vi "INTELLIFAUCET Need Adjustment PID.vi"(1 "GPM reading":dbl, 4 "GPM Target(3)":dbl, 5 "Error In":errorcluster, 10 "State":T1, 12 "TEMP,FLOW":T2=enum."FLOW") -> (13 "PI Output":dbl, 17 "Control Variable (Temp/GPM) Output":dbl, 18 "Micro Amp":i32, 19 "Error Out":errorcluster)   [LabVIEW 2023]
uses:
  Type Definitions/INTELLIFAUCT Temp Flow.ctl
  Type Definitions/HEWH Purge Draw.ctl
  <vilib>/addons/control/pid/NI_PID_autopid.lvlib
panel:
  in  "MV1:":dbl(slide)=15.081495361740814 scale=-100.0..100.0
  # "1.019811"
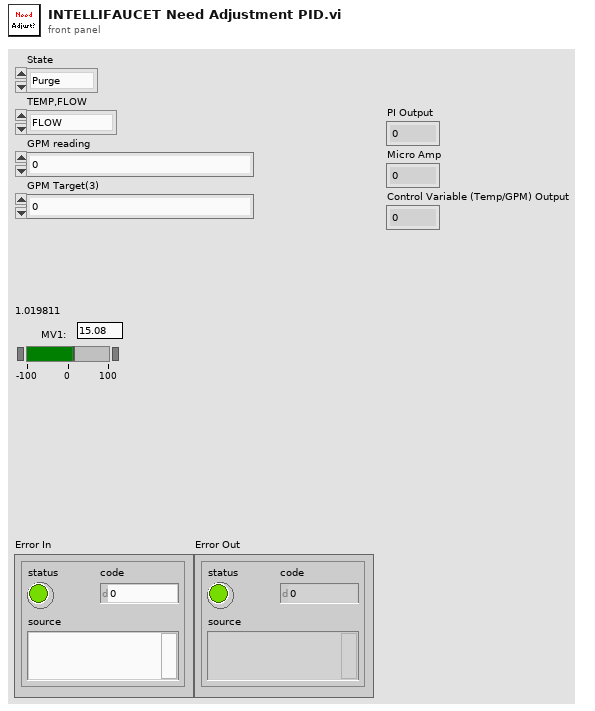
[diagram p1: front panel]
types:
  T1 = typedef "HEWH Purge Draw.ctl" = enum16{"Purge", "Draw"}
  T2 = typedef "INTELLIFAUCT Temp Flow.ctl" = enum8{"TEMP", "FLOW", "Prop Valve"}
  T3 = cluster{"process gain":dbl, "time constant (s)":dbl, "delay time (s)":dbl}
  T4 = cluster{"type of controller":u16, "time constant factor":dbl, "step amplitude":dbl}
  T5 = cluster{"proportional gain (Kc)":dbl, "integral time (Ti, min)":dbl, "derivative time (Td, min)":dbl}
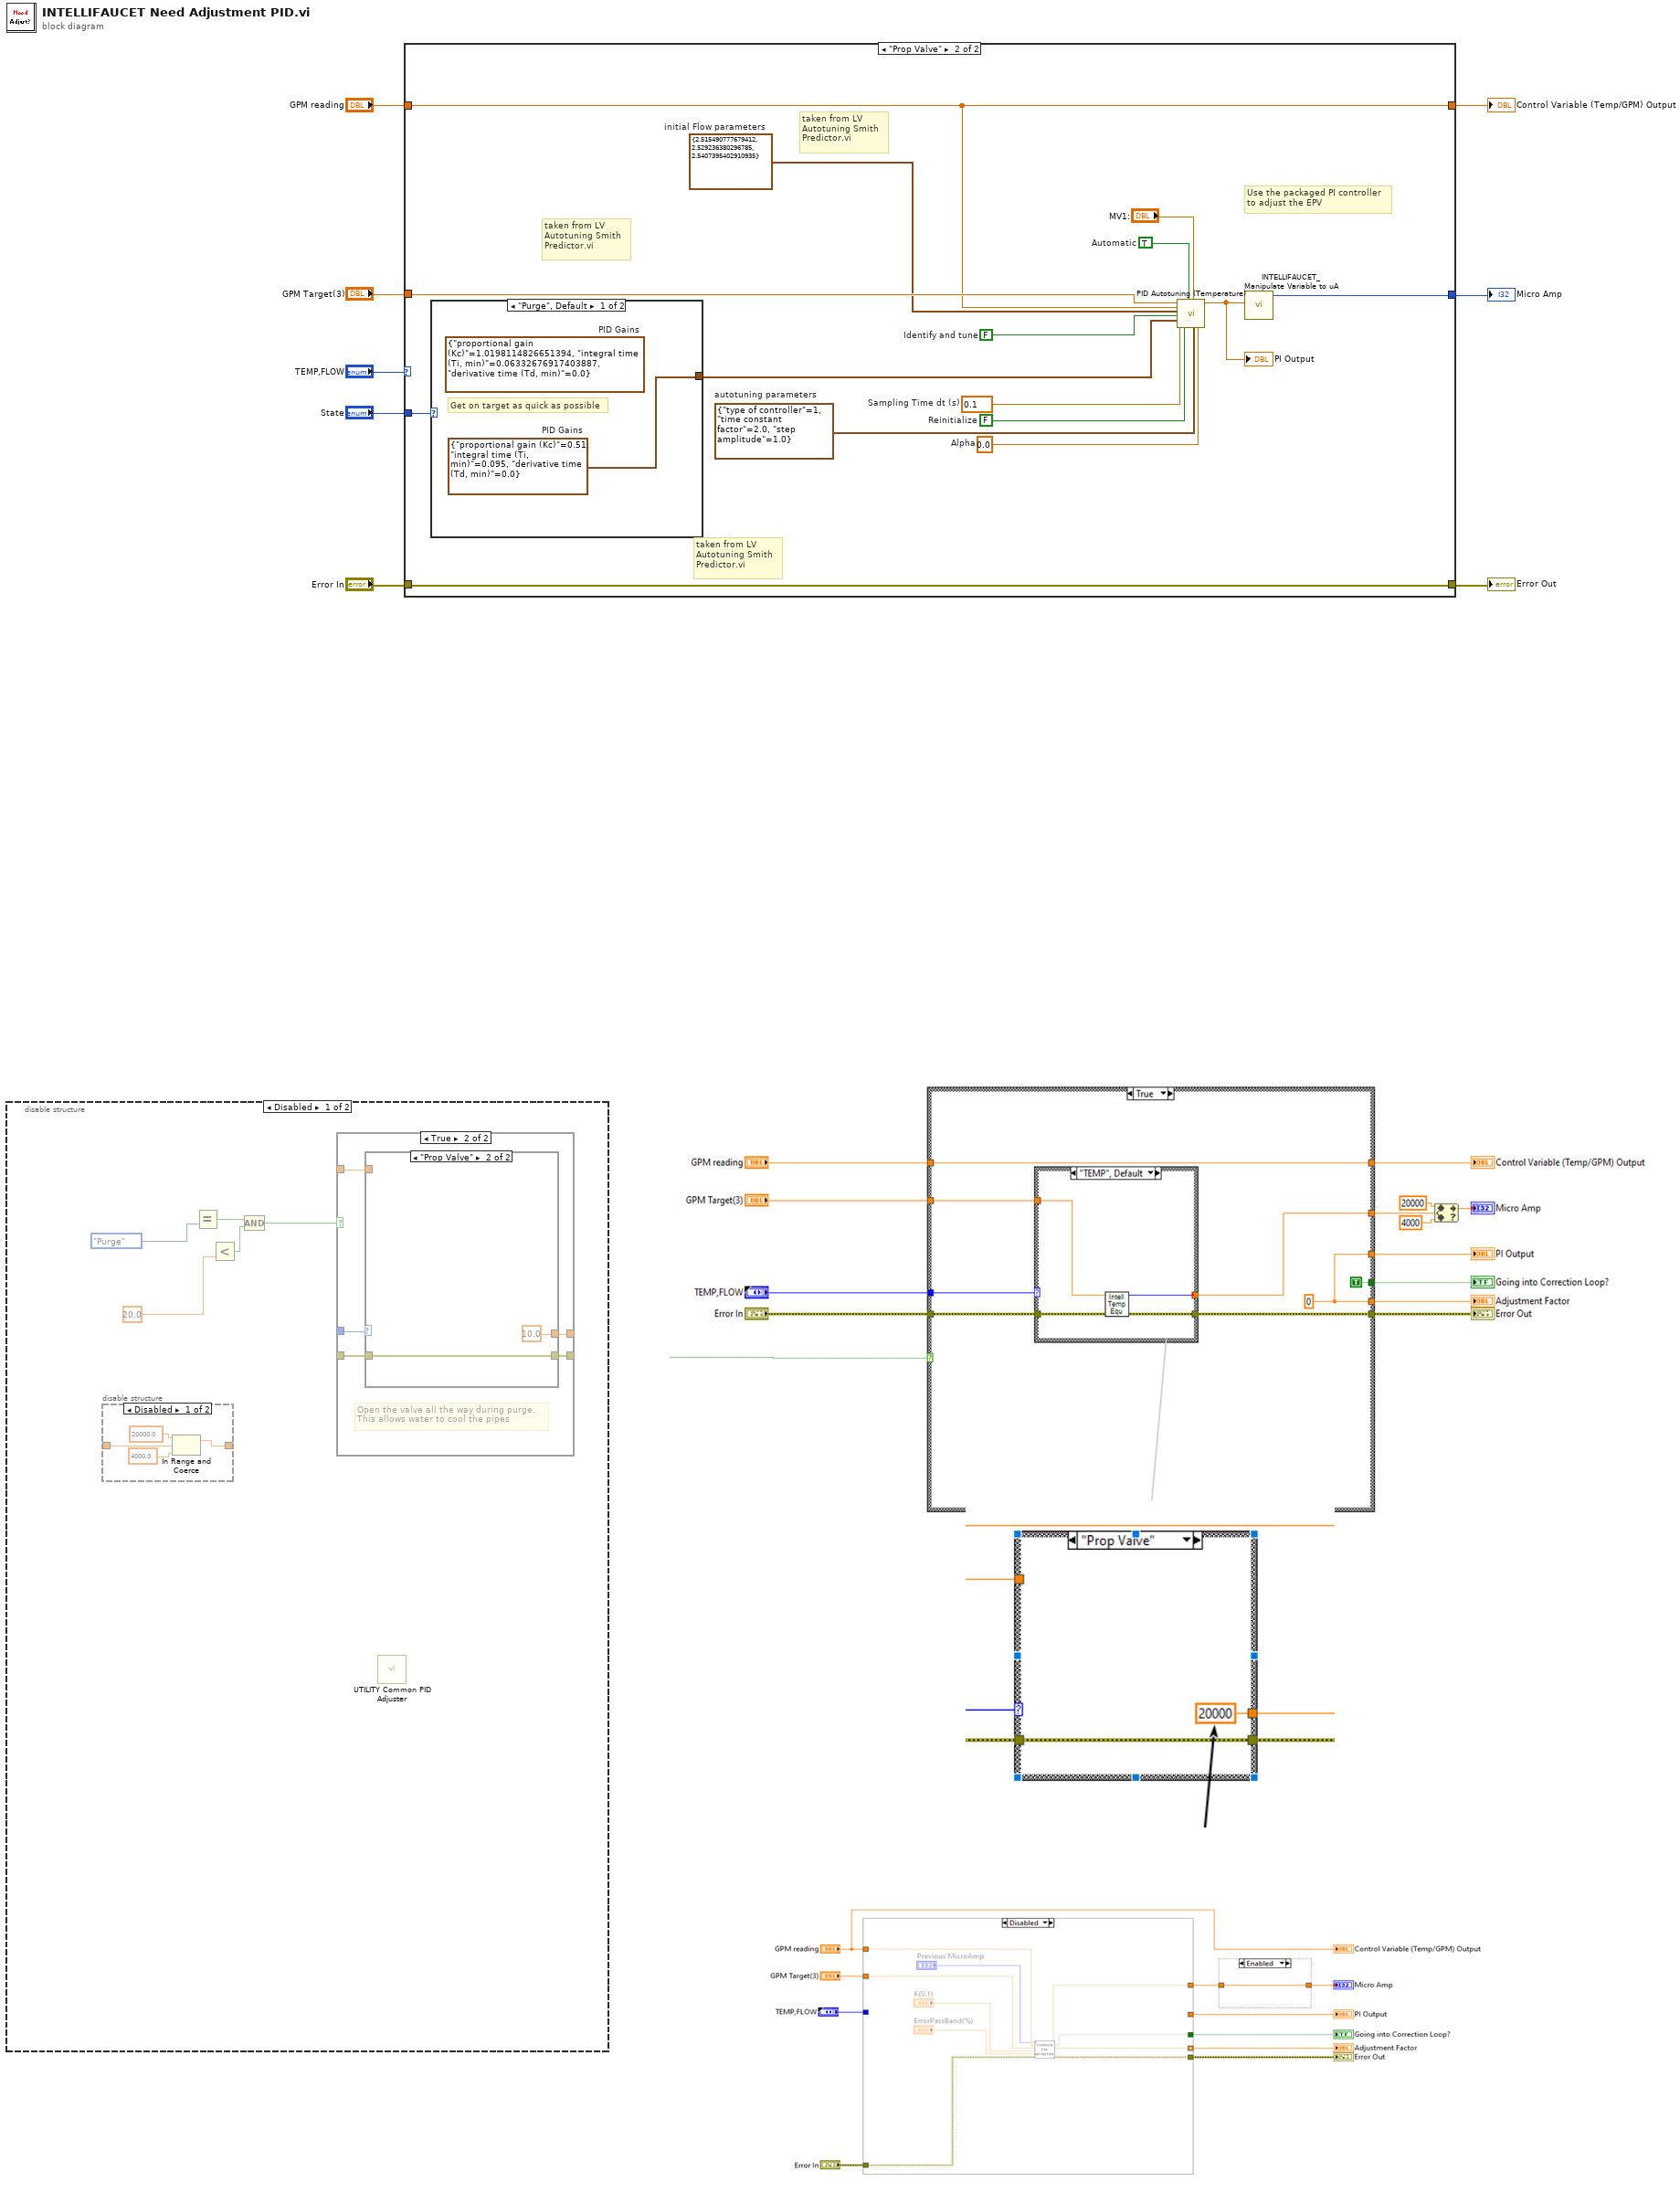
[diagram p0: block diagram]
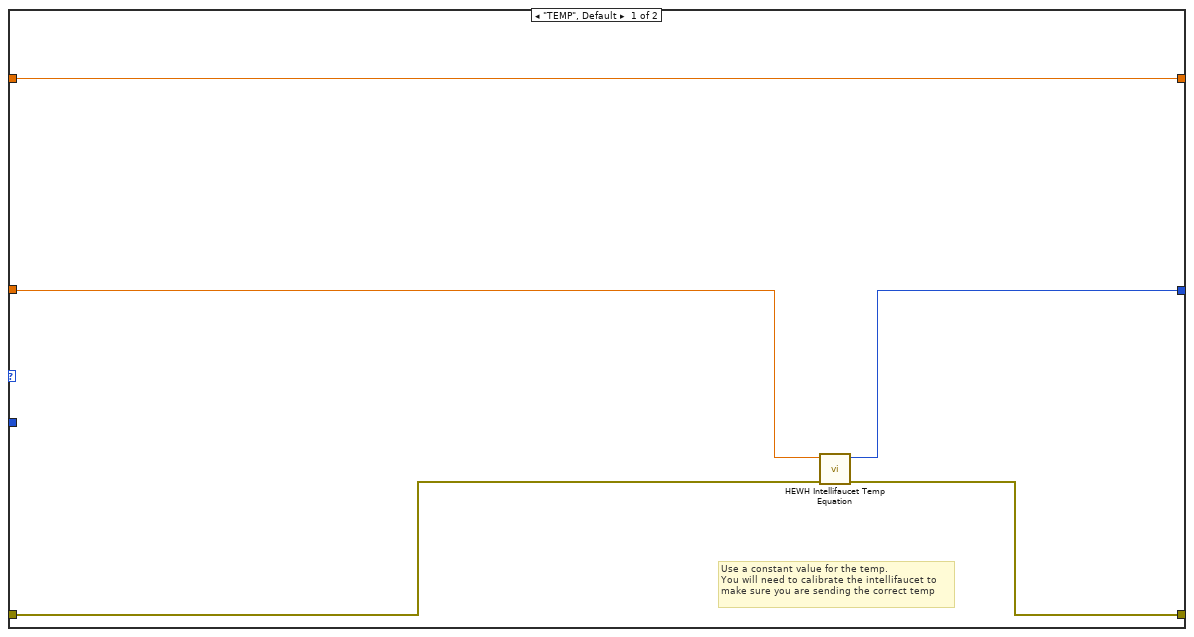
[diagram p2: hidden frame]
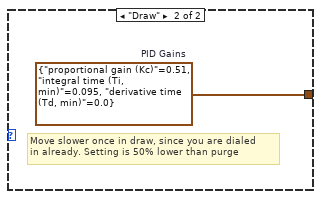
[diagram p3: hidden frame]
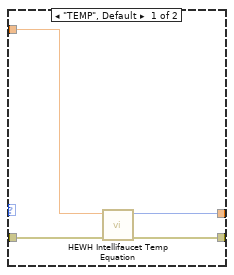
[diagram p6: hidden frame]
diagram:
  n1 = disable-structure shown="Disabled" {
    frame Disabled {
      n2 = disable-structure shown="Disabled" {
        disable-tunnel: [w17 w20] -> _
        disable-tunnel: _ -> [w16 w20]
        frame Disabled {
          n3 = In Range and Coerce(upper limit=20000.0, x=w16, lower limit=4000.0) -> (coerced(x)=w17:dbl)  [unwired: 1 out]
        }
        frame Enabled {
        }
      }
      n4 = Equal?(y=HEWH_Purge_Draw."Purge") -> (x=w15:T1, x = y?=w13:bool)
      n5 = Less?(y=20.0) -> (x=w12:dbl, x < y?=w10:bool)
      n6 = Compound Arithmetic op=AND(w13, w10) -> (w9:bool)
      n7 = case shown="True" w9 {
        tunnel: _ -> [_ w27]
        tunnel: _ -> [w21 w26]
        tunnel: [w21 w25] -> _
        tunnel: _ -> [w22 w24]
        tunnel: [w22 w23] -> _
        frame False {
        }
        frame True {
          # "Open the valve all the way during purge.\nThis allows water to cool the pipes"
          n8 = case shown="\"Prop Valve\"" w27 {
            tunnel: [w31 10.0 ("upper limit")] -> w23
            tunnel: w26 -> [w30 w32]
            tunnel: [w29 w32] -> w25
            tunnel: w24 -> [w28 _]
            frame "TEMP", Default {
              n9 = call "HEWH Intellifaucet Temp Equation.vi"("Error In"=w30, "Temp/GPM Target"=w28) -> ("Error Out"=w29:errorcluster, "Temp uA"=w31:i32)  [unwired: 7 in, 1 out]
            }
            frame "Prop Valve" {
            }
          }
        }
      }
      n10 = call "UTILITY Common PID Adjuster.vi"() -> ()  [unwired: 16 in, 4 out]
    }
    frame Enabled {
    }
  }
  n11 = case shown="\"Prop Valve\"" "TEMP,FLOW" {
    tunnel: [w34 w40] -> w8
    tunnel: "GPM Target(3)" -> [w36 w52]
    tunnel: [w35 w42] -> w6
    tunnel: "Error In" -> [w38 w41]
    tunnel: [w37 w41] -> w3
    tunnel: "GPM reading" -> [w34 w40]
    tunnel: "State" -> [_ w39]
    frame "TEMP", Default {
      # "Use a constant value for the temp.\nYou will need to calibrate the intellifaucet to\nmake sure you are sending the correct temp"
      n12 = call "HEWH Intellifaucet Temp Equation.vi"("Error In"=w38, "Temp/GPM Target"=w36) -> ("Error Out"=w37:errorcluster, "Temp uA"=w35:i32)  [unwired: 7 in, 1 out]
    }
    frame "Prop Valve" {
      w46 = T3 {"process gain"=2.515490777679412, "time constant (s)"=2.529236380296785, "delay time (s)"=2.5407395402910935}  # initial Flow parameters
      w47 = 0.1  # Sampling Time dt (s)
      w49 = TRUE  # Automatic
      w44 = FALSE  # Identify and tune
      w50 = FALSE  # Reinitialize
      w51 = T4 {"type of controller"=1, "time constant factor"=2.0, "step amplitude"=1.0}  # autotuning parameters
      w43 = 0.0  # Alpha
      # "taken from LV\nAutotuning Smith\nPredictor.vi"
      # "taken from LV\nAutotuning Smith\nPredictor.vi"
      # "taken from LV\nAutotuning Smith\nPredictor.vi"
      # "Use the packaged PI controller\nto adjust the EPV"
      n13 = case shown="\"Purge\", Default" w39 {
        tunnel: [w54 w55] -> w45
        frame "Purge", Default {
          w54 = T5 {"proportional gain (Kc)"=0.51, "integral time (Ti, min)"=0.095, "derivative time (Td, min)"=0.0}  # PID Gains
          (unwired) T5 {"proportional gain (Kc)"=1.0198114826651394, "integral time (Ti, min)"=0.06332676917403887, "derivative time (Td, min)"=0.0}  # PID Gains
          # "Get on target as quick as possible"
        }
        frame "Draw" {
          w55 = T5 {"proportional gain (Kc)"=0.51, "integral time (Ti, min)"=0.095, "derivative time (Td, min)"=0.0}  # PID Gains
          # "Move slower once in draw, since you are dialed\nin already. Setting is 50% lower than purge"
        }
      }
      n14 = call <vilib>:"PID Autotuning (Temperature).vi"("desired temperature"=w52, "measured temperature"=w40, "plant parameters in"=w46, "autotune? (F)"=w44, "PID gains in"=w45, "dt (s)"=w47, "reinitialize? (F)"=w50, "auto? (T)"=w49, "manual control"="MV1:", "autotuning parameters"=w51, "alpha"=w43) -> ("output"=w53:dbl)  [unwired: 5 in, 3 out]
      "PI Output" <- w53
      n15 = call "INTELLIFAUCET_Manipulate Variable to uA.vi"("MV"=w53) -> ("4-20uA Output"=w42:i32)  [unwired: 10 in]
    }
  }
  "Error Out" <- w3
  "Micro Amp" <- w6
  "Control Variable (Temp/GPM) Output" <- w8
